vi "Insert Lines Into Occupancy Grid.vi"(8 "Scale":dbl=0.1, 9 "Resolution":i32, 11 "Lines In":T1(array[cluster]) {"End Point"."Y" format="%.2f"; "End Point"."X" format="%.2f"; "Start Point"."Y" format="%.2f"; "Start Point"."X" format="%.2f"}) -> (0 "XY":cluster{dbl[], dbl[]}, 3 "M":dbl[](array[numeric]))   [LabVIEW 2012]
uses:
  <vilib>/Analysis/1siggen.llb/Ramp Pattern by Delta.vi
  <vilib>/Analysis/1siggen.llb/Ramp Pattern by Samples.vi
  <vilib>/Analysis/NI_AALBase.lvlib
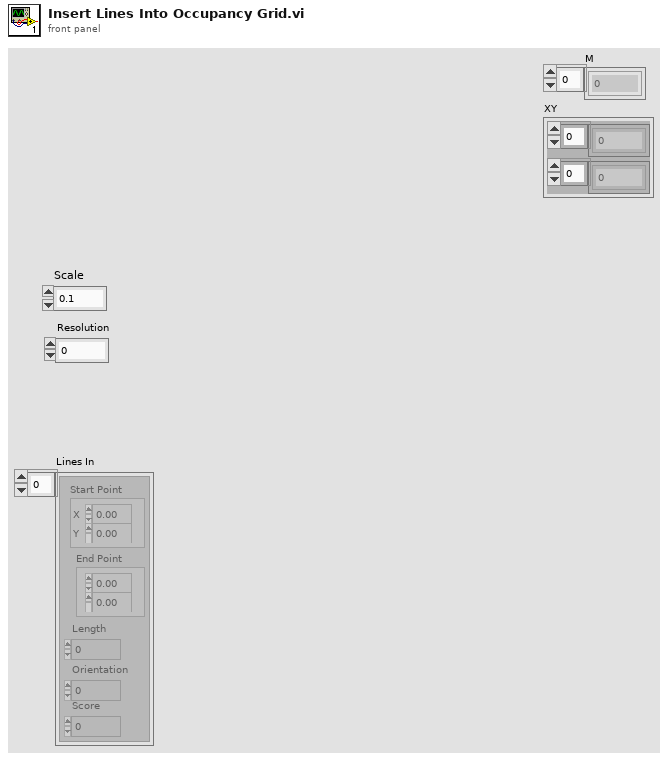
[diagram p1: front panel]
types:
  T1 = cluster{"Start Point":cluster{"X":sgl, "Y":sgl}, "End Point":cluster{"X":sgl, "Y":sgl}, "Length":dbl, "Orientation":dbl, "Score":dbl}[]
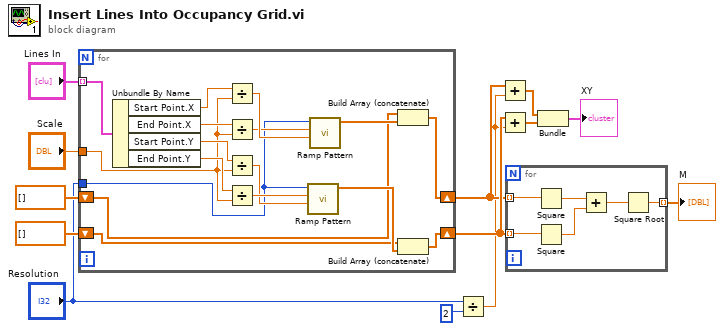
[diagram p0: block diagram]
diagram:
  n1 = for {
    tunnel: "Scale" -> [w14]
    tunnel: "Lines In" -> [w30] mode=indexing
    tunnel: "Resolution" -> [w21]
    shift-right: [w20] -> w3
    shift-left: dbl[] [] -> [w15]
    shift-right: [w18] -> w7
    shift-left: dbl[] [] -> [w16]
    n2 = Unbundle By Name(w30) -> ("Start Point.X"=w29:sgl, "End Point.X"=w26:sgl, "Start Point.Y"=w28:sgl, "End Point.Y"=w27:sgl)
    n3 = Divide(x=w29, y=w14) -> (x/y=w25:dbl)
    n4 = Divide(x=w26, y=w14) -> (x/y=w24:dbl)
    n5 = Divide(x=w28, y=w14) -> (x/y=w22:dbl)
    n6 = Divide(x=w27, y=w14) -> (x/y=w23:dbl)
    n7 = call-poly <vilib>:"Ramp Pattern.vi"("start"=w22, "end"=w23, "delta"=w21) -> ("Ramp Pattern"=w17:dbl[])  [unwired: 6 in, 2 out]
    n8 = call-poly <vilib>:"Ramp Pattern.vi"("start"=w25, "end"=w24, "samples"=w21) -> ("Ramp Pattern"=w19:dbl[])  [unwired: 7 in, 1 out]
    n9 = Build Array (concatenate)(w15, w19) -> (w20:dbl[])
    n10 = Build Array (concatenate)(w16, w17) -> (w18:dbl[])
  }
  n11 = Divide(x="Resolution", y=2) -> (x/y=w2:dbl)
  n12 = Add(x=w3, y=w2) -> (x+y=w1:dbl[])
  n13 = Add(x=w7, y=w2) -> (x+y=w4:dbl[])
  n14 = for {
    tunnel: w3 -> [w36] mode=indexing
    tunnel: w7 -> [w35] mode=indexing
    tunnel: [w31] -> w9 mode=indexing
    n15 = Square(x=w36) -> (x^2=w34:dbl)
    n16 = Square(x=w35) -> (x^2=w33:dbl)
    n17 = Add(x=w34, y=w33) -> (x+y=w32:dbl)
    n18 = Square Root(x=w32) -> (sqrt(x)=w31:dbl)
  }
  "M" <- w9
  n19 = Bundle(w1, w4) -> (→"XY":cluster{dbl[], dbl[]})  [unwired: 1 in]
